vi "Update_TimesweepDone_listbox.vi"(2 "new array":dbl[][](array[numeric])) -> (0 "New listbox":string[](array[string]))   [LabVIEW 2018]
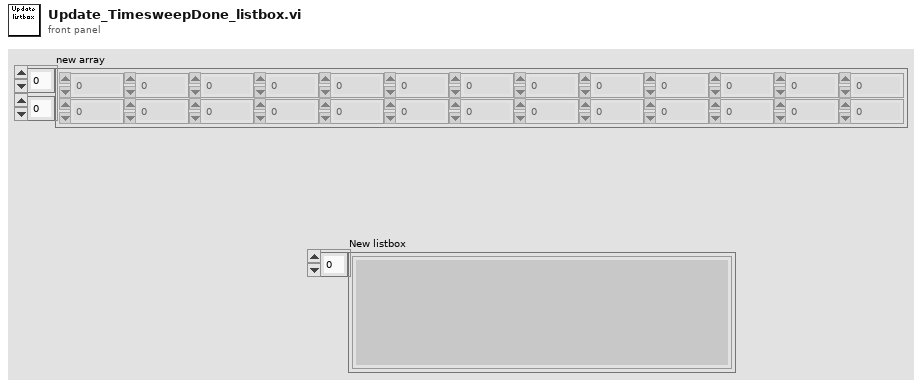
[diagram p1: front panel]
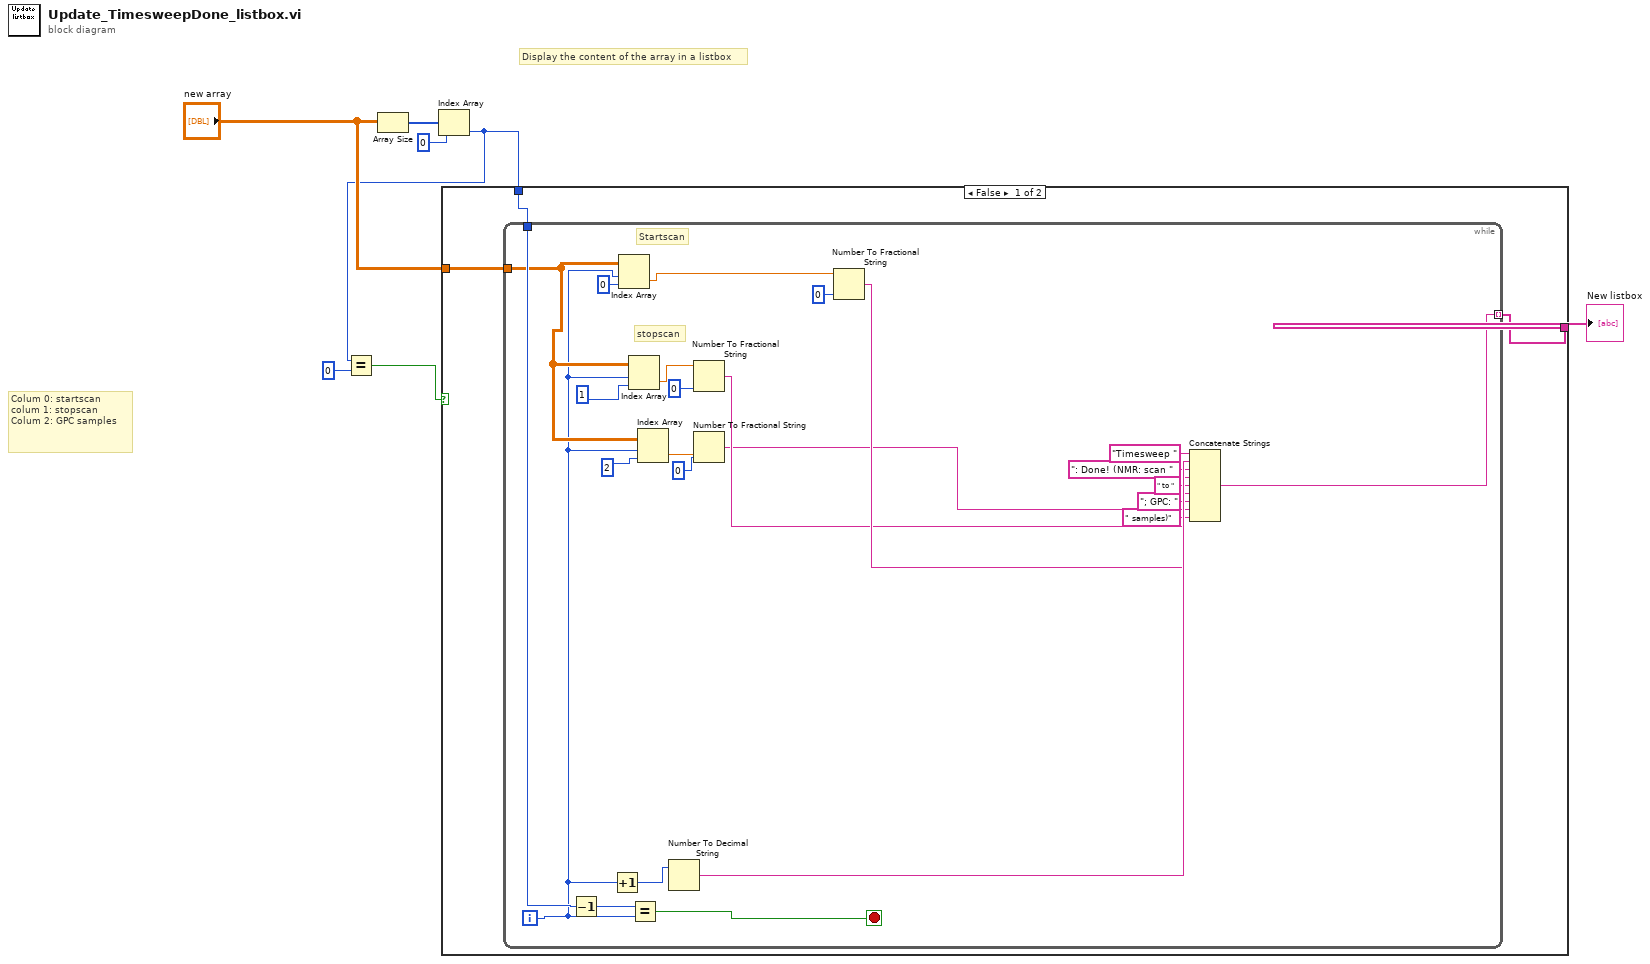
[diagram p0: block diagram]
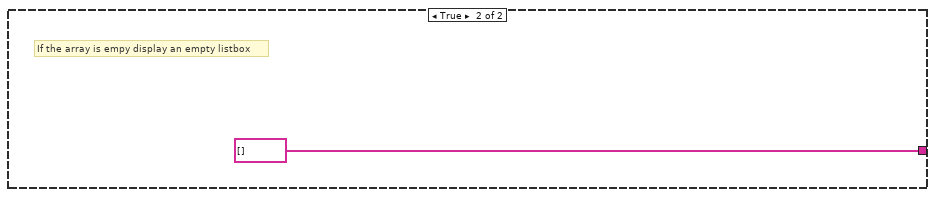
[diagram p2: hidden frame]
diagram:
  # "Colum 0: startscan\ncolum 1: stopscan\nColum 2: GPC samples"
  # "Display the content of the array in a listbox"
  n1 = Array Size(array="new array") -> (size(s)=w7:i32[])
  n2 = Index Array(array=w7, index=0) -> (element=w3:i32)
  n3 = Equal?(x=w3, y=0) -> (x = y?=w1:bool)
  n4 = case shown="False" w1 {
    tunnel: "new array" -> [w10 _]
    tunnel: w3 -> [w9 _]
    tunnel: [w8 string[] []] -> w4
    frame False {
      n5 = while {
        tunnel: w10 -> [w24]
        tunnel: w9 -> [w30]
        tunnel: [w25] -> w8 mode=indexing
        i -> [w23]
        stop <- w35 stop-if-true
        # "stopscan"
        # "Startscan"
        n6 = Decrement(x=w30) -> (x-1=w31:i32)
        n7 = Increment(x=w23) -> (x+1=w34:i32)
        n8 = Index Array(array=w24, index (row)=w23, index (col)=0 ("disabled index (col)")) -> (element=w22:dbl)
        n9 = Index Array(array=w24, index (row)=w23, index (col)=1 ("disabled index (col)")) -> (element=w20:dbl)
        n10 = Equal?(x=w31, y=w23) -> (x = y?=w35:bool)
        n11 = Index Array(array=w24, index (row)=w23, index (col)=2 ("disabled index (col)")) -> (element=w27:dbl)
        n12 = Number To Decimal String(number=w34) -> (decimal integer string=w18:string)  [unwired: 1 in]
        n13 = Number To Fractional String(number=w20, precision (6)=i16 0) -> (F-format string=w14:string)  [unwired: 2 in]
        n14 = Number To Fractional String(number=w27, precision (6)=i16 0) -> (F-format string=w12:string)  [unwired: 2 in]
        n15 = Number To Fractional String(number=w22, precision (6)=i16 0) -> (F-format string=w16:string)  [unwired: 2 in]
        n16 = Concatenate Strings("Timesweep " ("string"), w18, ": Done! (NMR: scan " ("string"), w16, " to " ("string"), w14, "; GPC: " ("string"), w12, " samples)" ("string")) -> (w25:string)
      }
    }
    frame True {
      # "If the array is empy display an empty listbox"
    }
  }
  "New listbox" <- w4
